vi "AjusteLockIn.vi"() -> ()   [LabVIEW 2018]
panel:
  in  "stop 3":bool
  out "Amplitud lockin":dbl[](graph)
  out "Frecuencia":dbl format="%#_5g"
  in  "stop":bool
  out "indicador":string
  out "error out":errorcluster
  in  "error in (no error)":errorcluster
  out "Cerca":bool
  out "Distancia Nano Z Act.":dbl
  out "limite":bool
  in  "stop 2":bool
  out "FFT":cluster{"f0":dbl, "df":dbl, "magnitude":dbl[]}[](graph) caption="fft"
  out "Amplitud":dbl[](graph)
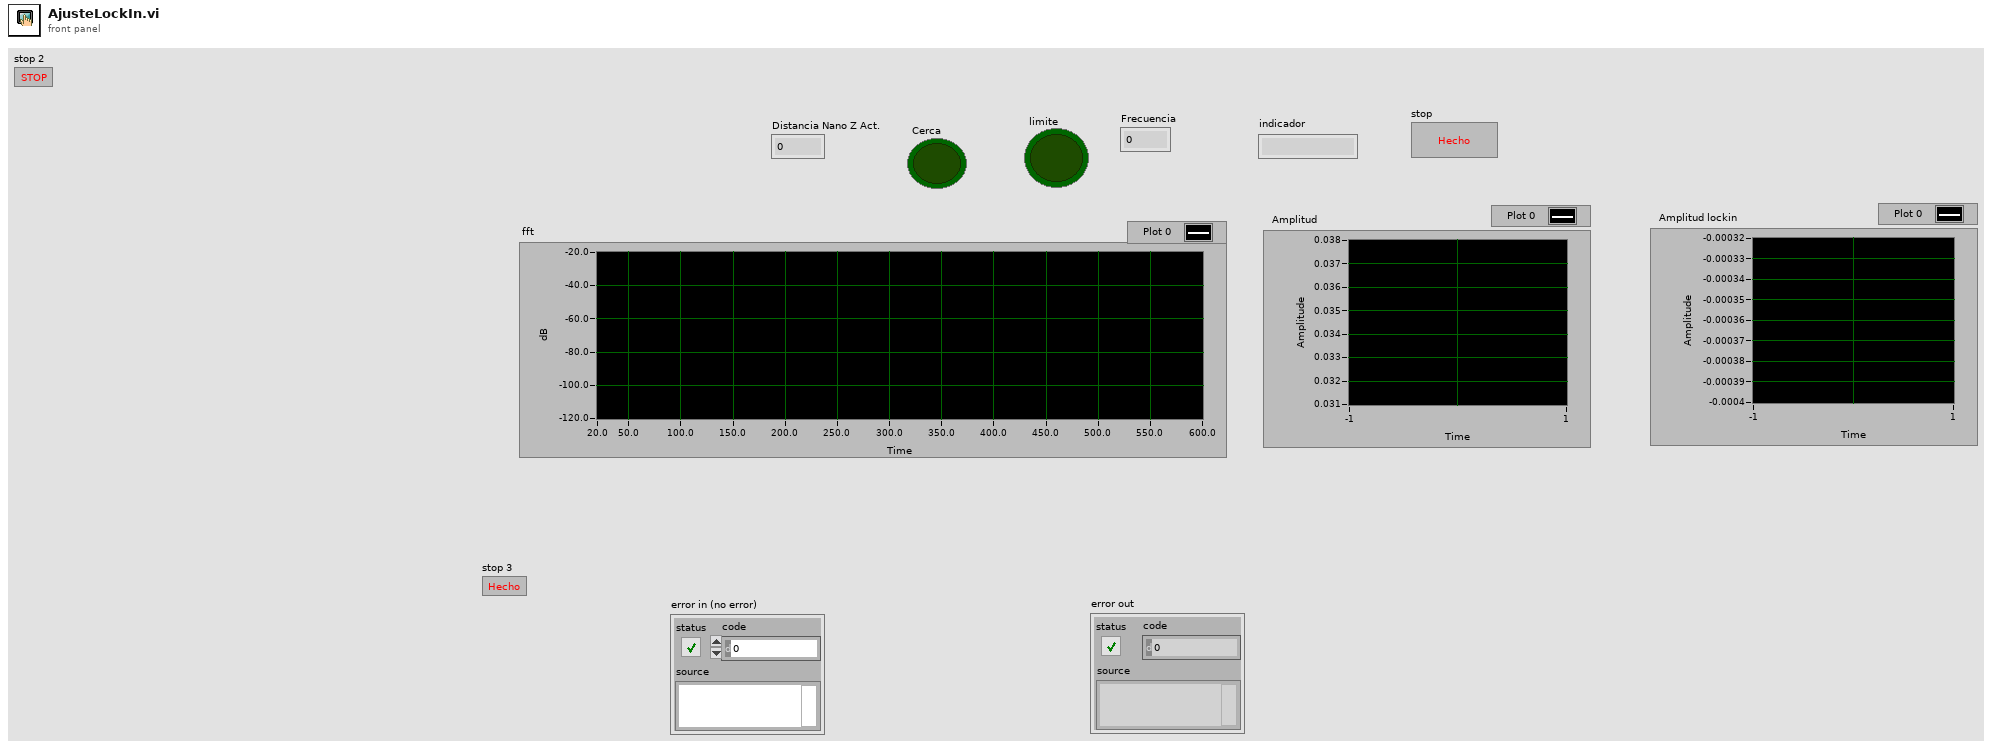
[diagram p1: front panel]
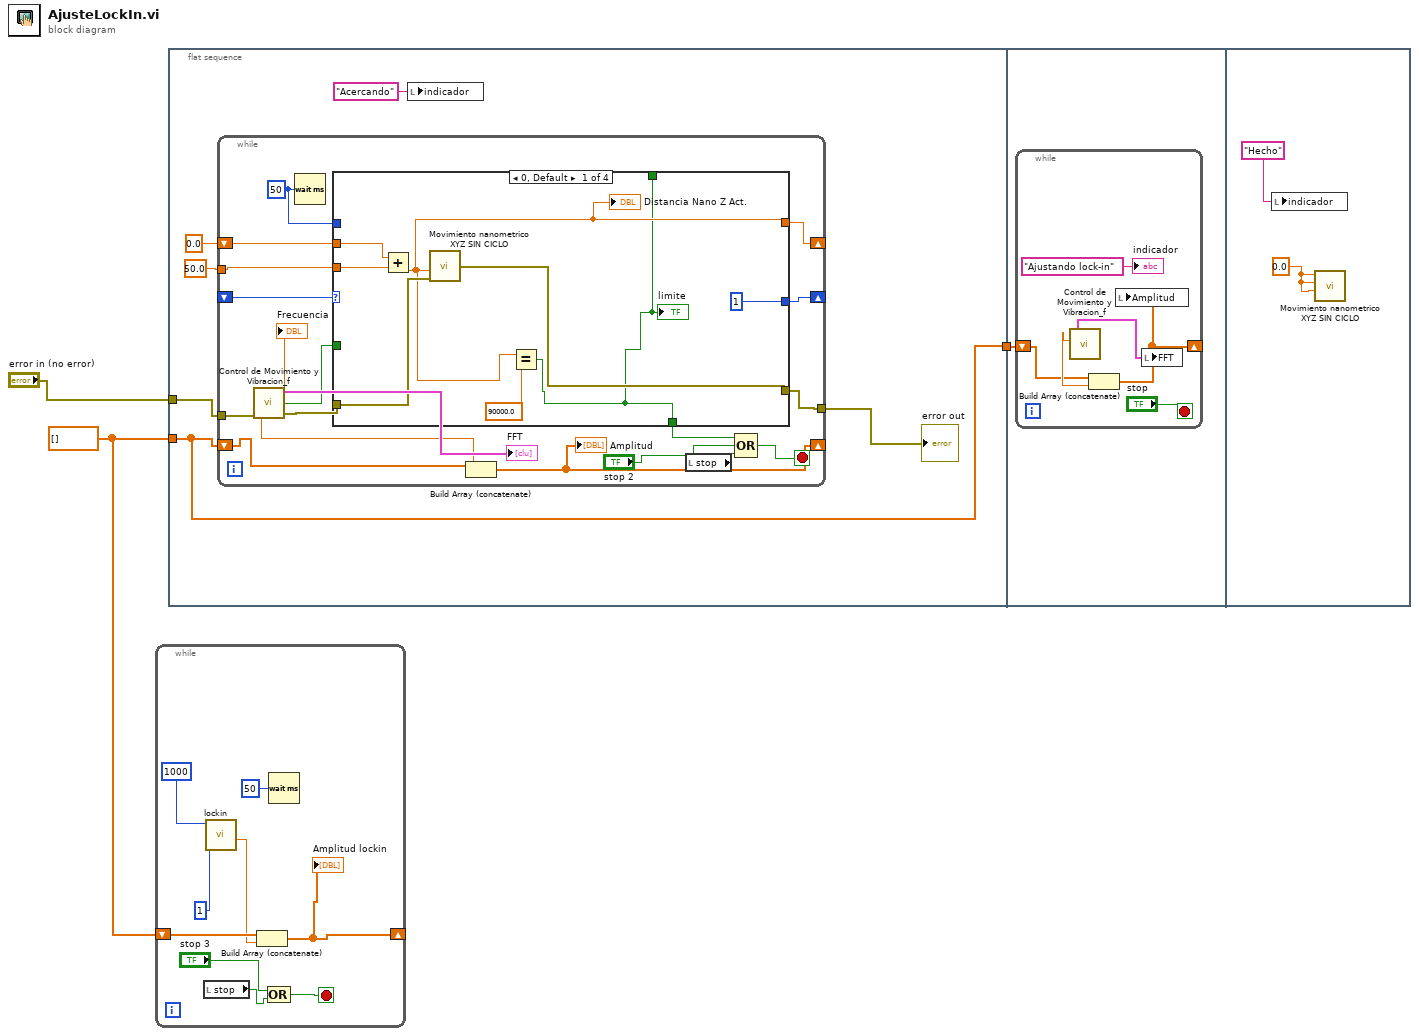
[diagram p0: block diagram]
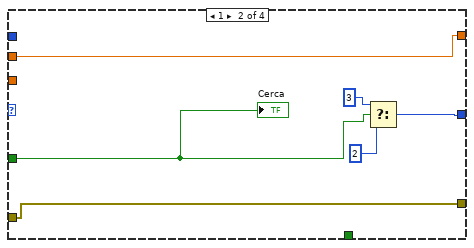
[diagram p2: hidden frame]
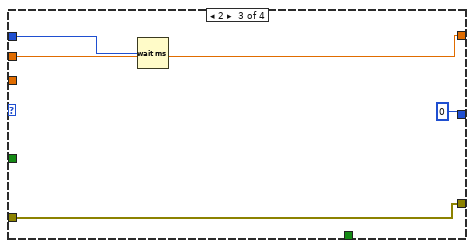
[diagram p3: hidden frame]
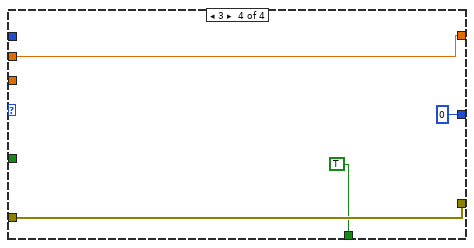
[diagram p4: hidden frame]
diagram:
  w1 = dbl[] []
  n1 = while {
    shift-right: [w7] -> _
    shift-left: w1 -> [w12]
    stop <- w5 stop-if-true
    n2 = local read "stop"() -> (w4:bool)
    n3 = call "lockin.vi"("NUMERO DE MED."=1, "milliseconds to wait"=u32 1000) -> ("Prom. Voltaje"=w11:dbl)  [unwired: 7 in, 2 out]
    n4 = Build Array (concatenate)(w12, w11) -> (w7:dbl[])
    "Amplitud lockin" <- w7
    n5 = Compound Arithmetic op=OR("stop 3", w4) -> (w5:bool)
    n6 = Wait (ms)(milliseconds to wait=u32 50) -> ()  [unwired: 1 out]
  }
  n7 = flat-sequence {
    tunnel: w1 -> [w14]
    tunnel: "error in (no error)" -> [w16]
    tunnel: [w14] -> w2
    tunnel: w2 -> [w60]
    frame #0 {
      n8 = while {
        shift-right: [w31] -> _
        shift-left: _ -> [w37]
        tunnel: w16 -> [w36]
        tunnel: 50.0 -> [w34]
        shift-right: [w33] -> _
        shift-left: 0.0 -> [w35]
        tunnel: [w30] -> w15
        shift-right: [w21] -> _
        shift-left: w14 -> [w22]
        stop <- w26 stop-if-true
        w29 = u32 50 ("milliseconds to wait")
        n9 = call "Control de Movimiento y Vibracion_f.vi"("Error In"=w36) -> ("Error Out"=w32:errorcluster, "Muy cerca"=w24:bool, "Frecuencia"=→"Frecuencia":dbl, "A"=w23:dbl, "FFT"=→"FFT":cluster{"f0":dbl, "df":dbl, "magnitude":dbl[]}[])  [unwired: 1 in]
        n10 = Wait (ms)(milliseconds to wait=w29) -> ()  [unwired: 1 out]
        n11 = case shown="0, Default" w37 {
          tunnel: w35 -> [w45 w47 w52 w58]
          tunnel: w34 -> [w44 _ _ _]
          tunnel: [w39 w47 w52 w58] -> w33
          tunnel: w32 -> [w43 w48 w54 w59]
          tunnel: [1 w50 0 0] -> w31
          tunnel: [w41 w48 w54 w59] -> w30
          tunnel: w24 -> [_ w46 _ _]
          tunnel: w29 -> [_ _ w53 _]
          tunnel: [w38 _ _ TRUE] -> w28
          tunnel: [w38 _ _ _] -> _
          frame 0, Default {
            n12 = Add(x=w45, y=w44) -> (x+y=w39:dbl)
            "Distancia Nano Z Act." <- w39
            n13 = call "Movimiento nanometrico XYZ SIN CICLO.vi"("Error In"=w43, "Movimiento en Z"=w39) -> ("Error Out"=w41:errorcluster)  [unwired: 4 in]
            n14 = Equal?(x=w39, y=90000.0) -> (x = y?=w38:bool)
            "limite" <- w38
          }
          frame 1 {
            n15 = Select(t=3, s=w46, f=2) -> (s? t:f=w50:i32)
            "Cerca" <- w46
          }
          frame 2 {
            n16 = Wait (ms)(milliseconds to wait=w53) -> ()  [unwired: 1 out]
          }
          frame 3 {
          }
        }
        n17 = Build Array (concatenate)(w22, w23) -> (w21:dbl[])
        "Amplitud" <- w21
        n18 = local read "stop"() -> (w19:bool)
        n19 = Compound Arithmetic op=OR(w28, "stop 2", w19) -> (w26:bool)
      }
      "error out" <- w15
      n20 = local write "indicador"("Acercando" ("indicador")) -> ()
    }
    frame #1 {
      n21 = while {
        shift-right: [w61] -> _
        shift-left: w60 -> [w62]
        stop <- "stop" stop-if-true
        n22 = call "Control de Movimiento y Vibracion_f.vi"() -> ("A"=w63:dbl, "FFT"=w64:cluster{"f0":dbl, "df":dbl, "magnitude":dbl[]}[])  [unwired: 2 in, 3 out]
        n23 = Build Array (concatenate)(w62, w63) -> (w61:dbl[])
        n24 = local write "Amplitud"(w61) -> ()
        n25 = local write "FFT"(w64) -> ()
        "indicador" <- "Ajustando lock-in" ("indicador")
      }
    }
    frame #2 {
      w68 = 0.0
      n26 = local write "indicador"("Hecho") -> ()
      n27 = call "Movimiento nanometrico XYZ SIN CICLO.vi"("Movimiento en Z"=w68, "Movimiento en Y"=w68, "Movimiento en X"=w68) -> ()  [unwired: 3 in, 1 out]
    }
  }
